vi "FROG_main.vi"() -> ()   [LabVIEW 2013]
panel:
  out "Fit Trace 2":dbl[][](graph)
  in  "Max Iterations":u16=250
  in  "Threshold":dbl=2.0 format="%_3e"
  out "Recovered Spectrum/Phase":cluster{ext[], dbl[]}[](graph)
  out "Retrieved Signal":cluster{ext[], "Gaussian noise pattern":dbl[]}(graph)
  out "RMS Error":dbl format="RMS = %#_3e"
  out "Error Log":dbl(graph)
  out "Iteration Count":i32
  out "Fit Trace":dbl[][](graph)
  out "Experiments Trace":dbl[][](graph)
  in  "Path":path
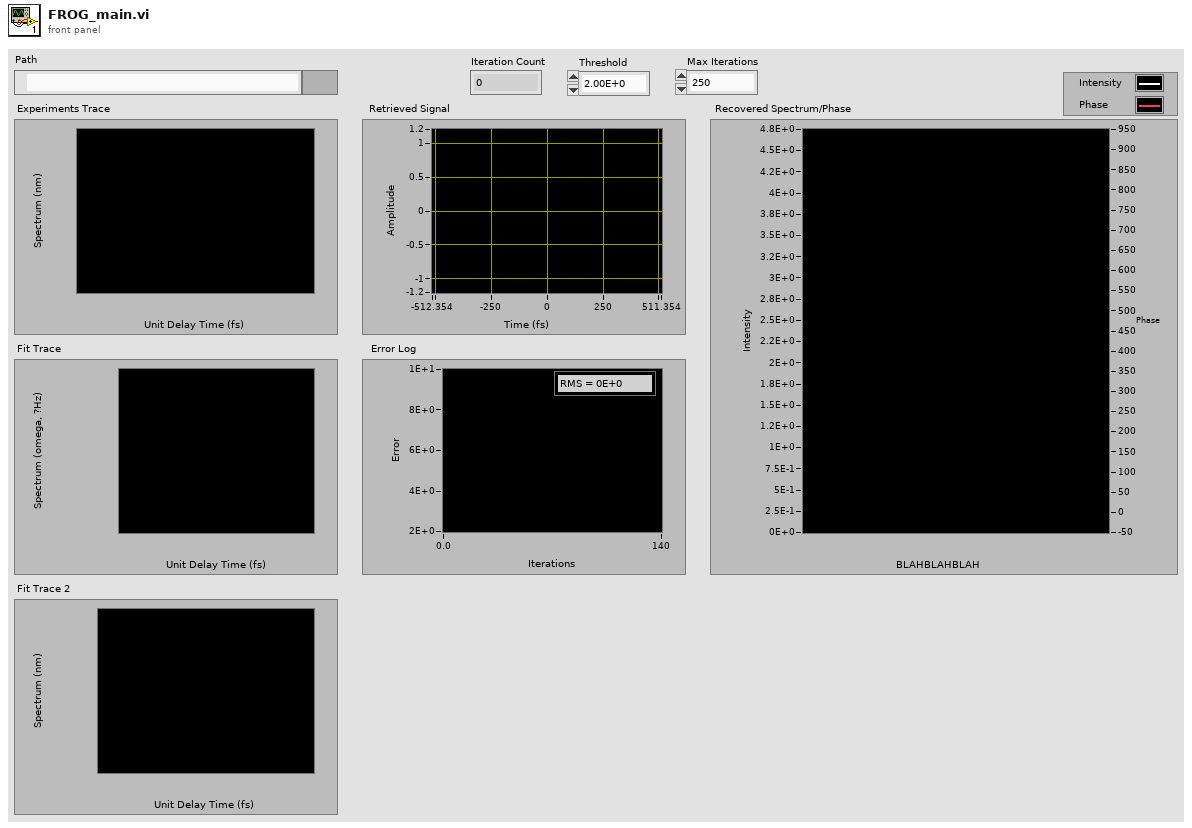
[diagram p1: front panel]
types:
  T1 = cluster{"Delay Temporal Resolution":u16, "Delay Spatial Resolution":u16}
  T2 = cluster{"Wavelength Max":dbl, "Wavelength Min":dbl, "Spectrum Resolution":u16}
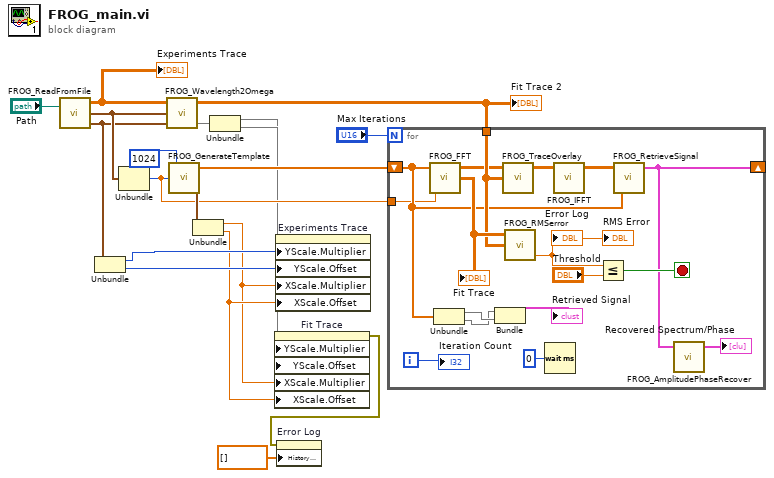
[diagram p0: block diagram]
diagram:
  n1 = call "FROG_ReadFromFile.vi"("File Path"="Path") -> ("Delay Info"=w4:T1, "Spectrum Info"=w5:T2, "Experiment Trace"=w7:dbl[][])  [unwired: 2 in]
  "Experiments Trace" <- w7
  n2 = Unbundle(w4) -> ("Delay Temporal Resolution"=w16:u16, "Delay Spatial Resolution"=w17:u16)
  n3 = Unbundle(w5) -> ("Wavelength Min"=w10:dbl, "Spectrum Resolution"=w19:u16)  [unwired: 1 out]
  n4 = call "FROG_Wavelength2Omega.vi"(3:w4, "Spectrum Info"=w5, "Experiment Trace"=w7) -> (0:w3, "Converted Trace"=w6:dbl[][])  [unwired: 1 out]
  "Fit Trace 2" <- w6
  n5 = call "FROG_GenerateTemplate.vi"("Delay Info"=w19, "Spectrum Info"=w10, 5:u16 1024 ("Signal Resolution")) -> ("Time Scale"=w15:cluster{"Time Multplier":dbl, "Time Offset":dbl}, "Noise Array"=w8:dbl[])  [unwired: 1 out]
  n6 = Unbundle(w15) -> ("Time Multplier"=w11:dbl, "Time Offset"=w14:dbl)
  n7 = Unbundle(w3) -> ("Spectrum Offset"=w1, "Spectrum Multplier"=w2)
  n8 = property on="Fit Trace" class="IntGraph (strict)"("YScale.Multiplier"=w2, "YScale.Offset"=w1, "XScale.Multiplier"=w11, "XScale.Offset"=w14) -> (error out=w12:errorcluster)  [unwired: 2 in, 1 out]
  n9 = property on="Experiments Trace" class="IntGraph (strict)"("YScale.Multiplier"=w16, "YScale.Offset"=w17, "XScale.Multiplier"=w11, "XScale.Offset"=w14) -> ()  [unwired: 2 in, 2 out]
  n10 = property on="Error Log" class="WFChart (strict)"(error in=w12, "History Data"=dbl[] []) -> ()  [unwired: 1 in, 2 out]
  n11 = for {
    N: "Max Iterations" -> [_]
    tunnel: w6 -> [w32]
    shift-right: [w21] -> _
    shift-left: w8 -> [w28]
    tunnel: w10 -> [w25]
    i -> [w37]
    stop <- w26 stop-if-true
    n12 = call "FROG_FFT.vi"("Time Delay Resolution"=w25, "Signal"=w28) -> ("Fit Trace"=w33:dbl[][], "Complex Electric Field"=w22:cdb[][])  [unwired: 2 in]
    "Fit Trace" <- w33
    n13 = Unbundle(w28) -> (w31, w30)
    n14 = Bundle(w30, w31) -> (→"Retrieved Signal":cluster{void, void})  [unwired: 1 in]
    n15 = call "FROG_TraceOverlay.vi"("Experiment Trace"=w32, "Complex Electric Field"=w22) -> ("Overlayed Complex Electric Field"=w34:cdb[][])  [unwired: 3 in]
    n16 = call "FROG_RMSerror.vi"("Experiment Trace"=w32, "Fit Trace"=w33) -> ("Histogram RMS Error"=w24:dbl)  [unwired: 1 in, 2 out]
    "Error Log" <- w24
    "RMS Error" <- w24
    n17 = Wait (ms)(milliseconds to wait=u32 0) -> ()  [unwired: 1 out]
    n18 = call "FROG_IFFT.vi"("Overlayed Complex Electric Field"=w34) -> ("Traced Pulse"=w35:cdb[][])  [unwired: 4 in]
    n19 = Less Or Equal?(x=w24, y="Threshold") -> (x <= y?=w26:bool)
    n20 = call "FROG_RetrieveSignal.vi"("Signal Template"=w28, "Traced Pulse"=w35) -> ("Retrieved Signal"=w21:cluster{"Gaussian noise pattern":dbl[], ext[]})  [unwired: 3 in]
    n21 = call "FROG_AmplitudePhaseRecover.vi"("Generated Signal"=w21) -> ("Array"=→"Recovered Spectrum/Phase":cluster{ext[], dbl[]}[])  [unwired: 4 in]
    "Iteration Count" <- w37
  }
